vi "Subvi buffer input.vi"(2 "Buffers":refnum<k21>="AB0") -> ()   [LabVIEW 2017]
uses:
  GV FIFO timeout.vi
  <vilib>/rvi/interface/RandomDataEmulation/niFpgaRandomDataHandleErrors.vi
  <vilib>/rvi/DataTransferAndStorage/Container/Common/niFpgaContainerExecOnDevCompGetState.vi
  <vilib>/rvi/Emulation/niFpgaEmulationIsFPGAContextNoSignature.vi
  <vilib>/rvi/Emulation/niFpgaSctlEmulationGetInTimedLoop.vi
  <vilib>/rvi/errors/niFpgaSetErrorForExecOnDevCompSimple.vi
  <vilib>/rvi/eio/common/nirviEmuReportErrorAndStop.vi
  <vilib>/rvi/DataTransferAndStorage/Container/Common/niFpgaContainerGetUniqueNameForEmu.vi
  <vilib>/rvi/FIFO/Fifo_Resource/nirvififoEmulationSetSize.vi
  <vilib>/rvi/FIFO/Fifo_Resource/nirviFifoEmulationQueueMgr.vi
  <instcachedir>/0/nirviFifoEmulationQueueMgr_E5CAEC123FF24DC58D834DCA3CDAA9B5.lvgen/nirviFifoEmulationQueueMgr_E5CAEC123FF24DC58D834DCA3CDAA9B5_001.vi
  <vilib>/rvi/FIFO/Fifo_Resource/nirvififoEmulationDetermineInputValidOut.vi
  <vilib>/rvi/FIFO/Fifo_Resource/nirvififoEmulationCreateLock.vi
  <vilib>/rvi/Emulation/niFpgaProcessEmulError.vi
  <vilib>/rvi/FIFO/Fifo_Resource/nirvififoEmulationObtainLock.vi
  <vilib>/rvi/FIFO/Fifo_Resource/nirvififoEmulationReleaseLock.vi
  <vilib>/rvi/occurrence/nirviWaitOnOccurrenceBase.vi
  <vilib>/rvi/errors/nirviReportUnexpectedCaseInternalError.vi
  <vilib>/rvi/errors/nirviReportUnexpectedCaseInternalError (U32).vi
  <vilib>/Utility/error.llb/Clear Errors.vi
  <vilib>/rvi/DataTransferAndStorage/Container/XNode/niFpgaContainer.xnode
  <vilib>/rvi/interface/RandomDataEmulation/nirviRandomDataFpgaReadWriteTemplate.vi
  <vilib>/rvi/FIFO/Fifo_Resource/niFpgaFifoEmulationRefIn.vi
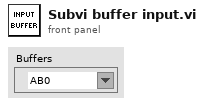
[diagram p1: front panel]
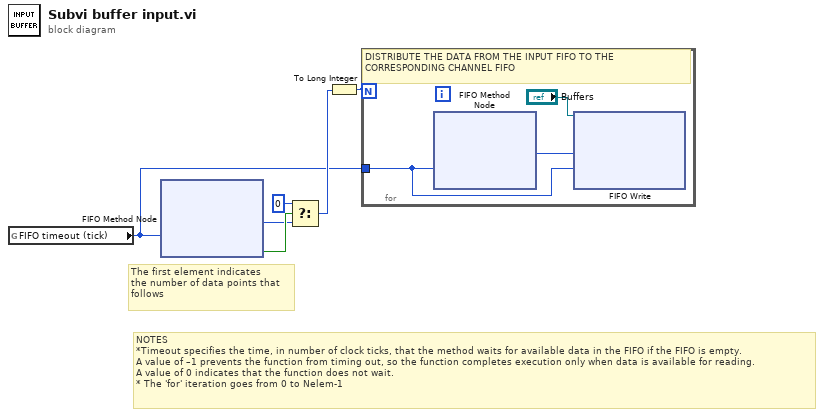
[diagram p0: block diagram]
diagram:
  # "The first element indicates\nthe number of data points that\nfollows"
  # "NOTES\n*Timeout specifies the time, in number of clock ticks, that the method waits for available data in the FIFO if the FIFO is empty.\nA value of –1 prevents the function from timing out, so the function completes execution only when data is available for reading.\nA value of 0 indicates that the function does not wait.\n* The 'for' iteration goes from 0 to Nelem-1"
  n1 = global read "GV FIFO timeout.vi" "FIFO timeout (tick)"() -> (w3:i32)
  n2 = xnode ("FIFO Method Node")("Timeout"=w3) -> ("Element"=w1:u32, "Timed Out?"=w2:bool)  [unwired: 1 in, 1 out]
  n3 = Select(t=u32 0, s=w2, f=w1) -> (s? t:f=w4:u32)
  n4 = To Long Integer(number=w4) -> (32bit integer=w5:i32)
  n5 = for {
    N: w5 -> [_]
    tunnel: w3 -> [w7]
    # "DISTRIBUTE THE DATA FROM THE INPUT FIFO TO THE CORRESPONDING CHANNEL FIFO"
    n6 = xnode ("FIFO Method Node")("Timeout"=w7) -> ("Element"=w8:u32)  [unwired: 1 in, 2 out]
    n7 = xnode ("FIFO Write")("Element"=w8, "Timeout"=w7, "FIFO In"="Buffers") -> ()  [unwired: 2 out]
  }
